vi "Test Process Lifecycle States.vi"(8 "error in (no error)":errorcluster, 11 "Process Test In":refnum<class "Process Test.lvclass">) -> (0 "error out":errorcluster, 3 "Process Test Out":refnum<class "Process Test.lvclass">)   [LabVIEW 2020, in "Process Test.lvclass"]
uses:
  Process Test.lvclass
  C:/Program Files (x86)/National Instruments/LabVIEW 2020/vi.lib/Asteme/LUnit/Test Case.lvclass
  Framework/Process/Public/TypeDefs/Lifecycle State.ctl
  Framework/Process/Process.lvclass/Process.ctl
  <vilib>/Asteme/LUnit/Test Case.lvclass/Test Case.ctl
  <vilib>/Asteme/LUnit/LUnit Assertion Result.lvclass/LUnit Assertion Result.ctl
  <vilib>/Utility/error.llb/Clear Errors.vi
  <vilib>/Asteme/LUnit/Palette/Fail.vi
  <vilib>/Asteme/LUnit/Palette/Pass.vi
  <vilib>/Asteme/LUnit/Set Assertion Type.vi
  Framework/Process/Private/SubVIs/Wait for finish.vi
  Framework/Process/Protected/Messaging/Enqueue Message.vi
  Framework/Process/Private/SubVIs/Set Lifecycle State.vi
  <vilib>/Asteme/LUnit/Add test result.vi
  <vilib>/Asteme/LUnit/LUnit Write Passed.vi
  <vilib>/Asteme/LUnit/LUnit Get Test Case.vi
  <vilib>/Asteme/LUnit/LUnit Write Message.vi
  <vilib>/Asteme/LUnit/LUnit Write Description.vi
  <vilib>/Asteme/LUnit/LUnit Write Assertion Type.vi
  <vilib>/AdvancedString/1D String Array to Delimited String.vi
  <vilib>/Asteme/LUnit/Read Test Case Name.vi
  <vilib>/Asteme/LUnit/Assertion Result/LUnit Get Test Name.vi
  <vilib>/Utility/error.llb/Error Cluster From Error Code.vi
  <vilib>/Asteme/LUnit/LUnit Assertion Result.lvclass
  Framework/Process/Process.lvclass
  <vilib>/Asteme/LUnit/Test Case.lvclass
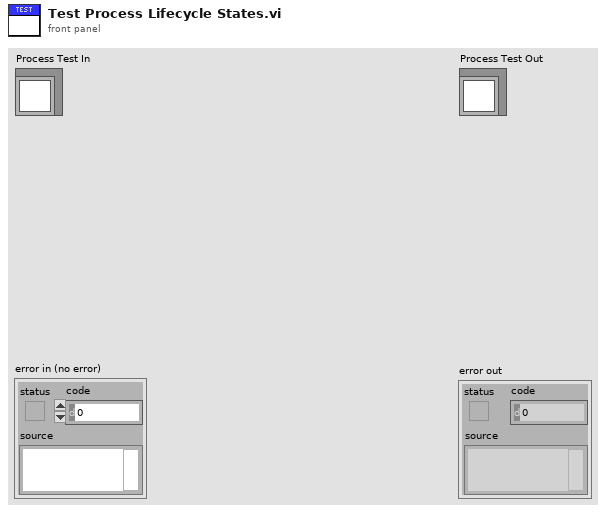
[diagram p1: front panel]
types:
  T1 = typedef "Process.lvclass/Lifecycle State.ctl" = enum16{"Uninitialized", "Initialized", "Started", "Running", "Stopped", "Finished"}
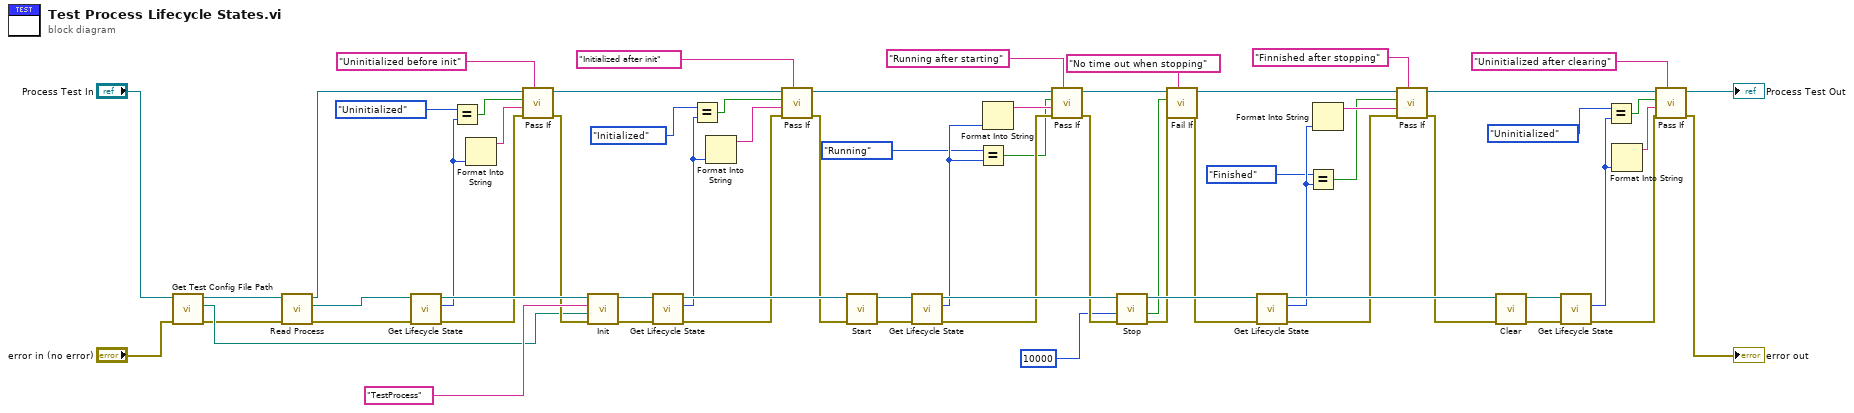
[diagram p0: block diagram]
diagram:
  n1 = call-dynamic "Get Test Config File Path.vi"("error in (no error)"="error in (no error)", "Base Class Test in"="Process Test In") -> ("error out"=w10:errorcluster, "Test config path"=w29:path, "Base Class Test out"=w12:refnum<class "Process Test.lvclass">)  [unwired: 7 in]
  n2 = call "Read Process.vi"("error in (no error)"=w10, "Process Test in"=w12) -> ("error out"=w9:errorcluster, "Process.lvclass"=w11:refnum<class "Process.lvclass">, "Process Test out"=w7:refnum<class "Process Test.lvclass">)  [unwired: 7 in]
  n3 = call "Get Lifecycle State.vi"("error in (no error)"=w9, "Process In"=w11) -> ("error out"=w50:errorcluster, "Lifecycle State"=w25:T1, "Process Out"=w66:refnum<class "Process.lvclass">)  [unwired: 6 in, 1 out]
  n4 = Equal?(x=Lifecycle_State."Uninitialized" ("Lifecycle State"), y=w25) -> (x = y?=w24:bool)
  n5 = Format Into String(w25) -> (resulting string=w23:string)  [unwired: 3 in, 1 out]
  n6 = call <vilib>:"Pass If.vi"("Description"="Uninitialized before init", "error in (no error)"=w50, "Message"=w23, "Pass?"=w24, "Test Case In"=w7) -> ("error out"=w49:errorcluster, "Test Case Out"=w54:refnum<class "Process Test.lvclass">)  [unwired: 5 in]
  n7 = call-dynamic "Init.vi"("error in (no error)"=w49, "Config File Path"=w29, "Name"="TestProcess", "Process In"=w66) -> ("error out"=w64:errorcluster, "Process Out"=w65:refnum<class "Process.lvclass">)  [unwired: 6 in]
  n8 = call "Get Lifecycle State.vi"("error in (no error)"=w64, "Process In"=w65) -> ("error out"=w48:errorcluster, "Lifecycle State"=w28:T1, "Process Out"=w63:refnum<class "Process.lvclass">)  [unwired: 6 in, 1 out]
  n9 = Equal?(x=Lifecycle_State."Initialized" ("Lifecycle State"), y=w28) -> (x = y?=w27:bool)
  n10 = Format Into String(w28) -> (resulting string=w26:string)  [unwired: 3 in, 1 out]
  n11 = call <vilib>:"Pass If.vi"("Description"="Initialized after init", "error in (no error)"=w48, "Message"=w26, "Pass?"=w27, "Test Case In"=w54) -> ("error out"=w47:errorcluster, "Test Case Out"=w53:refnum<class "Process Test.lvclass">)  [unwired: 5 in]
  n12 = call "Start.vi"("error in (no error)"=w47, "Process In"=w63) -> ("error out"=w61:errorcluster, "Process Out"=w62:refnum<class "Process.lvclass">)  [unwired: 8 in]
  n13 = call "Get Lifecycle State.vi"("error in (no error)"=w61, "Process In"=w62) -> ("error out"=w46:errorcluster, "Lifecycle State"=w36:T1, "Process Out"=w60:refnum<class "Process.lvclass">)  [unwired: 6 in, 1 out]
  n14 = Equal?(x=Lifecycle_State."Running" ("Lifecycle State"), y=w36) -> (x = y?=w18:bool)
  n15 = Format Into String(w36) -> (resulting string=w35:string)  [unwired: 3 in, 1 out]
  n16 = call <vilib>:"Pass If.vi"("Description"="Running after starting", "error in (no error)"=w46, "Message"=w35, "Pass?"=w18, "Test Case In"=w53) -> ("error out"=w45:errorcluster, "Test Case Out"=w52:refnum<class "Process Test.lvclass">)  [unwired: 5 in]
  n17 = call "Stop.vi"("error in (no error)"=w45, "timeout in ms (-1)"=10000, "Process In"=w60) -> ("error out"=w14:errorcluster, "timed out?"=w16:bool, "Process Out"=w59:refnum<class "Process.lvclass">)  [unwired: 6 in]
  n18 = call <vilib>:"Fail If.vi"("Description"="No time out when stopping", "error in (no error)"=w14, "Fail?"=w16, "Test Case In"=w52) -> ("error out"=w13:errorcluster, "Test Case Out"=w17:refnum<class "Process Test.lvclass">)  [unwired: 6 in]
  n19 = call "Get Lifecycle State.vi"("error in (no error)"=w13, "Process In"=w59) -> ("error out"=w44:errorcluster, "Lifecycle State"=w33:T1, "Process Out"=w58:refnum<class "Process.lvclass">)  [unwired: 6 in, 1 out]
  n20 = Equal?(x=Lifecycle_State."Finished" ("Lifecycle State"), y=w33) -> (x = y?=w19:bool)
  n21 = Format Into String(w33) -> (resulting string=w32:string)  [unwired: 3 in, 1 out]
  n22 = call <vilib>:"Pass If.vi"("Description"="Finnished after stopping", "error in (no error)"=w44, "Message"=w32, "Pass?"=w19, "Test Case In"=w17) -> ("error out"=w43:errorcluster, "Test Case Out"=w51:refnum<class "Process Test.lvclass">)  [unwired: 5 in]
  n23 = call-dynamic "Clear.vi"("error in (no error)"=w43, "Process In"=w58) -> ("error out"=w56:errorcluster, "Process Out"=w57:refnum<class "Process.lvclass">)  [unwired: 8 in]
  n24 = call "Get Lifecycle State.vi"("error in (no error)"=w56, "Process In"=w57) -> ("error out"=w42:errorcluster, "Lifecycle State"=w21:T1)  [unwired: 6 in, 2 out]
  n25 = Equal?(x=Lifecycle_State."Uninitialized" ("Lifecycle State"), y=w21) -> (x = y?=w22:bool)
  n26 = Format Into String(w21) -> (resulting string=w20:string)  [unwired: 3 in, 1 out]
  n27 = call <vilib>:"Pass If.vi"("Description"="Uninitialized after clearing", "error in (no error)"=w42, "Message"=w20, "Pass?"=w22, "Test Case In"=w51) -> ("error out"=→"error out":errorcluster, "Test Case Out"=→"Process Test Out":refnum<class "Process Test.lvclass">)  [unwired: 5 in]
